vi "12bit_2sComplement.vi"   [LabVIEW 2012]
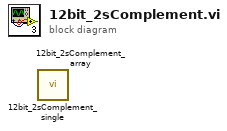
[diagram p0: block diagram]
diagram:
  n1 = call "12bit_2sComplement_single.vi"() -> ()  [unwired: 1 in, 1 out]
  n2 = call "12bit_2sComplement_array.vi"() -> ()  [unwired: 1 in, 1 out]
